vi "Alarma Bool.vi"() -> ()   [LabVIEW 2020]
panel:
  out "Texto 3":string
  out "Texto 2":string
  out "Texto 1":string
  out "Alarma 3":bool
  out "Alarma 2":bool
  out "Alarma 1":bool
  in  "Limite Minimo":u8(slide) scale=0.0..100.0
  in  "Limite MAXIMO":u8(slide) scale=0.0..100.0
  in  "TEMP 3":dbl(slide) scale=0.0..100.0
  in  "TEMP 2":dbl(slide) scale=0.0..100.0
  in  "TEMP 1":dbl(slide) scale=0.0..100.0
  # "ALARMA BOOLEANA"
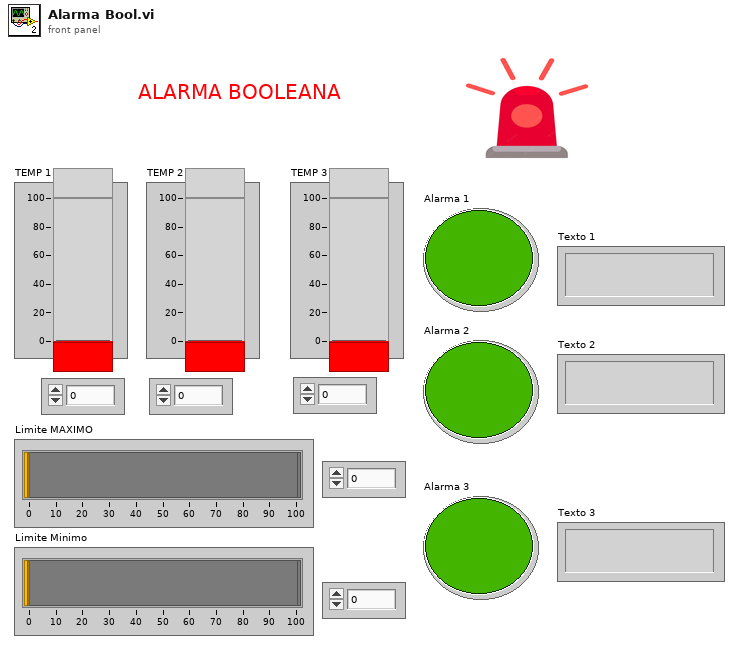
[diagram p1: front panel]
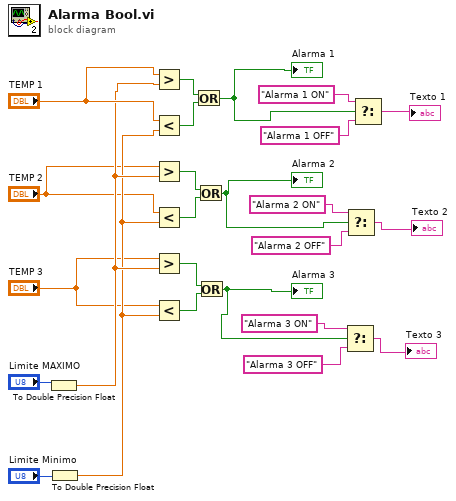
[diagram p0: block diagram]
diagram:
  n1 = To Double Precision Float(number="Limite MAXIMO") -> (double precision float=w21:dbl)
  n2 = To Double Precision Float(number="Limite Minimo") -> (double precision float=w20:dbl)
  n3 = Greater?(x="TEMP 1", y=w21) -> (0:w19:bool)
  n4 = Less?(x="TEMP 1", y=w20) -> (x < y?=w18:bool)
  n5 = Greater?(x="TEMP 2", y=w21) -> (0:w25:bool)
  n6 = Less?(x="TEMP 2", y=w20) -> (x < y?=w17:bool)
  n7 = Greater?(x="TEMP 3", y=w21) -> (0:w16:bool)
  n8 = Less?(x="TEMP 3", y=w20) -> (x < y?=w15:bool)
  n9 = Or(x=w19, y=w18) -> (x .or. y?=w12:bool)
  "Alarma 1" <- w12
  n10 = Or(x=w25, y=w17) -> (x .or. y?=w6:bool)
  "Alarma 2" <- w6
  n11 = Or(x=w16, y=w15) -> (x .or. y?=w5:bool)
  "Alarma 3" <- w5
  n12 = Select(t="Alarma 3 ON", s=w5, f="Alarma 3 OFF") -> (s? t:f=→"Texto 3":string)
  n13 = Select(t="Alarma 2 ON", s=w6, f="Alarma 2 OFF") -> (s? t:f=→"Texto 2":string)
  n14 = Select(t="Alarma 1 ON", s=w12, f="Alarma 1 OFF") -> (s? t:f=→"Texto 1":string)
